vi "FTW-Socket-Send.vi"(0 "FTW Socket":refnum<class "FTW-Socket.lvclass">, 5 "Message":string, 7 "Send Timeout":i32 format="%dmsec", 11 "error in":errorcluster) -> (4 "FTW Socket out":refnum<class "FTW-Socket.lvclass">, 6 "Timed out?":bool, 15 "error out":errorcluster)   [LabVIEW 2013, in "FTW-Socket.lvclass"]
uses:
  FTW-Socket.lvclass
  FTW-Socket.lvclass/FTW-Socket.ctl
panel:
  # "Inputs"
  # "Outputs"
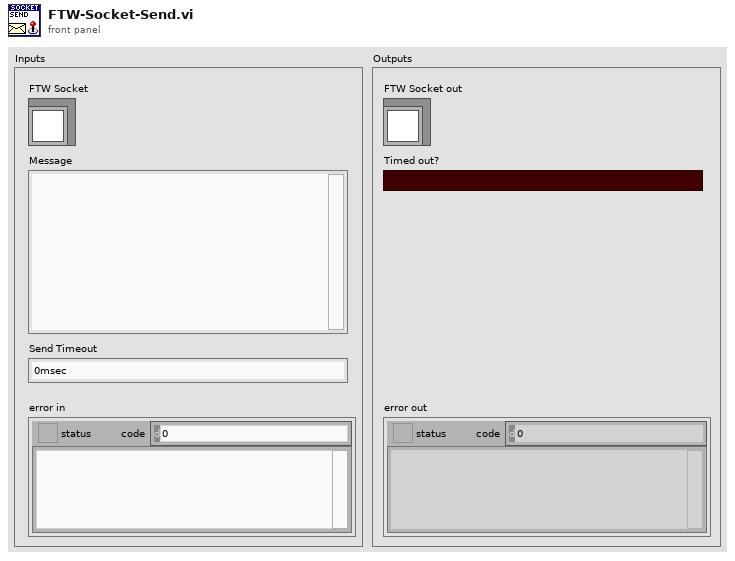
[diagram p1: front panel]
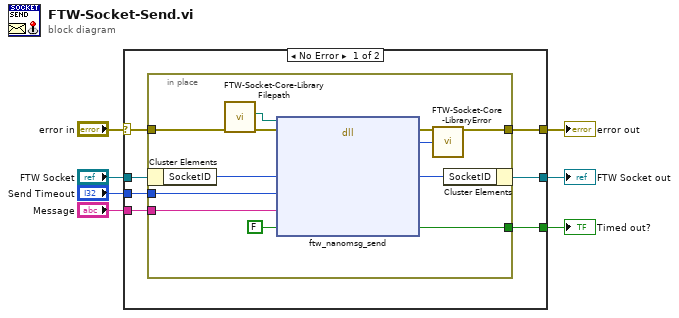
[diagram p0: block diagram]
diagram:
  n1 = case shown="No Error" "error in" {
    selector: "error in" -> [w11 w27]
    tunnel: "FTW Socket" -> [w14 w28]
    tunnel: "Message" -> [w13 _]
    tunnel: [w9 w27] -> w3
    tunnel: [w12 w28] -> w4
    tunnel: "Send Timeout" -> [w10 _]
    tunnel: [w8 _] -> w1
    frame No Error {
      n2 = in-place {
        in-place-border: w11 -> [w26]
        in-place-border: [w22] -> w9
        in-place-border: w10 -> [w19]
        in-place-border: w13 -> [w17]
        in-place-border: [w15] -> w8
        n3 = in-place-cluster #1(w14) -> ("SocketID"=w24:i64)
        n4 = call "FTW-Socket-Core-LibraryFilepath.vi"("error in"=w26) -> ("error out"=w20:errorcluster, "Library Filepath"=w21:path)  [unwired: 8 in, 1 out]
        n5 = dll-call lib="?" fn="ftw_nanomsg_send"(path in=w21, error in=w20, "SocketID"=w24, "Timeout"=w19, "Outgoing Message"=w17, "Timed out?"=FALSE) -> (error out=w25:errorcluster, "Return Value"=w18:i64, "SocketID"=w23:i64, "Timed out?"=w15:bool)  [unwired: 5 in, 1 out]
        n6 = call "FTW-Socket-Core-LibraryError.vi"("error in"=w25, "Return Value"=w18) -> ("error out"=w22:errorcluster)  [unwired: 13 in]
        n7 = in-place-cluster #1("SocketID"=w23) -> (w12:refnum<class "FTW-Socket.lvclass">)
      }
    }
    frame Error {
    }
  }
  "error out" <- w3
  "FTW Socket out" <- w4
  "Timed out?" <- w1
